vi "Coloring B-Scan Demo.vi"() -> ()   [LabVIEW 2012]
uses:
  LabVIEW/user.lib/SpectralRadar.llb/Color Enhancement Selection.ctl
  LabVIEW/user.lib/SpectralRadar.llb/Colorscheme Selection.ctl
  LabVIEW/user.lib/SpectralRadar.llb/Coloring Byteorder.ctl
  LabVIEW/user.lib/SpectralRadar.llb/Device Camera Preset Selection.ctl
  LabVIEW/user.lib/SpectralRadar.llb/Processing Parameter Int Selection.ctl
  LabVIEW/user.lib/SpectralRadar.llb/Probe Parameter Int Selection.ctl
  LabVIEW/user.lib/SpectralRadar.llb/Colored Data Export Format Selection.ctl
  LabVIEW/user.lib/SpectralRadar.llb/set Transposed Colored Scan Output.vi
  LabVIEW/user.lib/SpectralRadar.llb/set Scan Output.vi
  LabVIEW/user.lib/SpectralRadar.llb/Data.lvclass
  LabVIEW/user.lib/SpectralRadar.llb/OCT Device.lvclass
  LabVIEW/user.lib/SpectralRadar.llb/Probe.lvclass
  LabVIEW/user.lib/SpectralRadar.llb/Processing.lvclass
  LabVIEW/user.lib/SpectralRadar.llb/Raw Data.lvclass
  LabVIEW/user.lib/SpectralRadar.llb/Scan Pattern.lvclass
  LabVIEW/user.lib/SpectralRadar.llb/Coloring.lvclass
  LabVIEW/user.lib/SpectralRadar.llb/Colored Data.lvclass
  <vilib>/Analysis/NI_AALBase.lvlib
  <vilib>/Analysis/NI_AALPro.lvlib
  LabVIEW/user.lib/SpectralRadar.llb/LabVIEW Helper.lvlib
panel:
  in  "Save Button":bool
  in  "File Name":path
  in  "Display On/Off":bool
  in  "Range":dbl=1.0
  in  "Show Histogram":bool
  in  "Equalize":bool
  out "XY Graph 2":cluster{"X Values":dbl[], "Integral X":dbl[]}(graph)
  in  "Autoscale":bool
  out "XY Graph":T1(graph)
  in  "Color Table Selection":T2
  out "Averaged Frame Rate":dbl=6.134969234466553 format="%#_3g"
  out "Current Frame Rate":dbl=6.134969234466553 format="%#_3g"
  in  "Color Enhancement":T3
  in  "Boundries":cluster{sgl, sgl}(slide)={76.65738, 42.00557} scale=-20.0..120.0
  out "Image":T4(plugin-control)
  in  "stop":bool
  in  "AScans":i32=1024
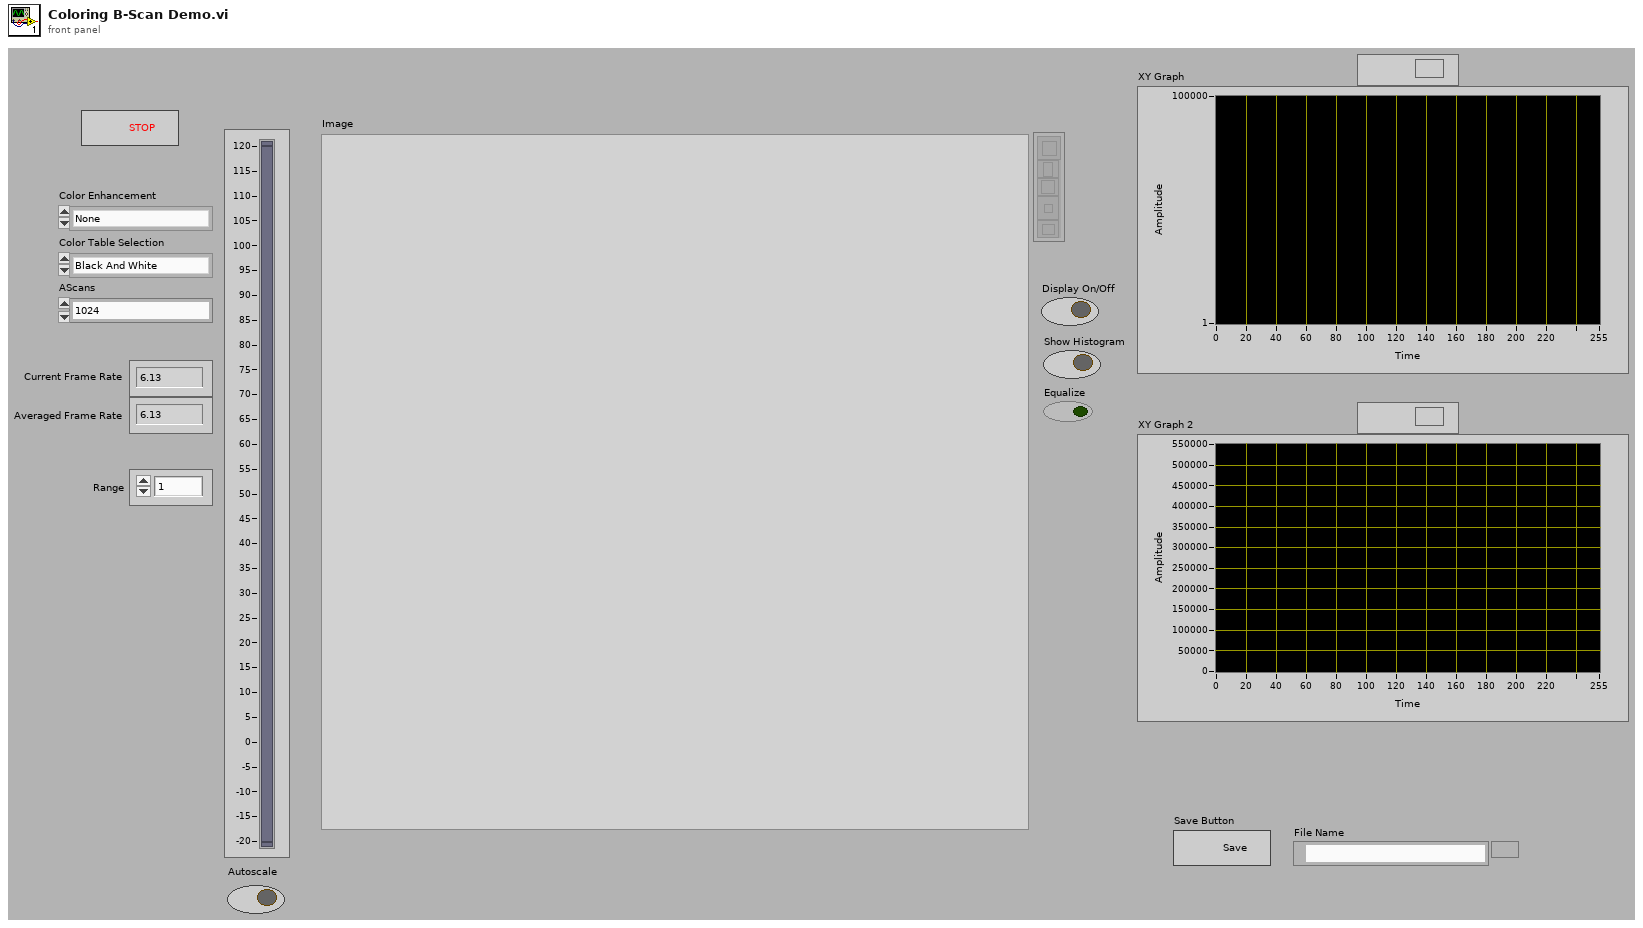
[diagram p1: front panel]
types:
  T1 = cluster{"X Values":dbl[], "Histogram: h(x)":i32[]}
  T2 = typedef "Coloring.lvclass/Colorscheme Selection.ctl" = enum16{"Black And White", "Inverted Black And White", "Color", "Black and Orange", "Black and Red", "Doppler Phase Coloring"}
  T3 = typedef "Coloring.lvclass/Color Enhancement Selection.ctl" = enum16{"None", "Sine", "Parable", "Cubic", "Square Root"}
  T4 = typedef "IMAQ Image.ctl" = refnum<image>
  T5 = typedef "Probe.lvclass/Probe Parameter Int Selection.ctl" = enum16{"Apodization Cycles", "Oversampling", "White Balance Auto", "Oversampling Slow Axis"}
  T6 = typedef "Processing.lvclass/Processing Parameter Int Selection.ctl" = enum32{"Spectrum Averaging", "A-Scan Averaging", "B-Scan Averaging", "Zero Padding", "Number of Threads", "Fourier Averaging"}
  T7 = typedef "OCT Device.lvclass/Device Camera Preset Selection.ctl" = enum16{"Default", "Preset 1", "Preset 2", "Preset 3"}
  T8 = typedef "Coloring.lvclass/Coloring Byteorder.ctl" = enum16{"RGBA32", "BGRA32", "ARGB32", ""}
  T9 = typedef "Image Type" = u32
  T10 = enum16{"Asynchronous Continuous", "Asynchronous Finite", "Synchronous"}
  T11 = typedef "Colored Data.lvclass/Colored Data Export Format Selection.ctl" = enum16{"SRM (Spectral Radar Metafile)", "RAW", "BMP", "PNG", "JPG", "PDF", "TIFF"}
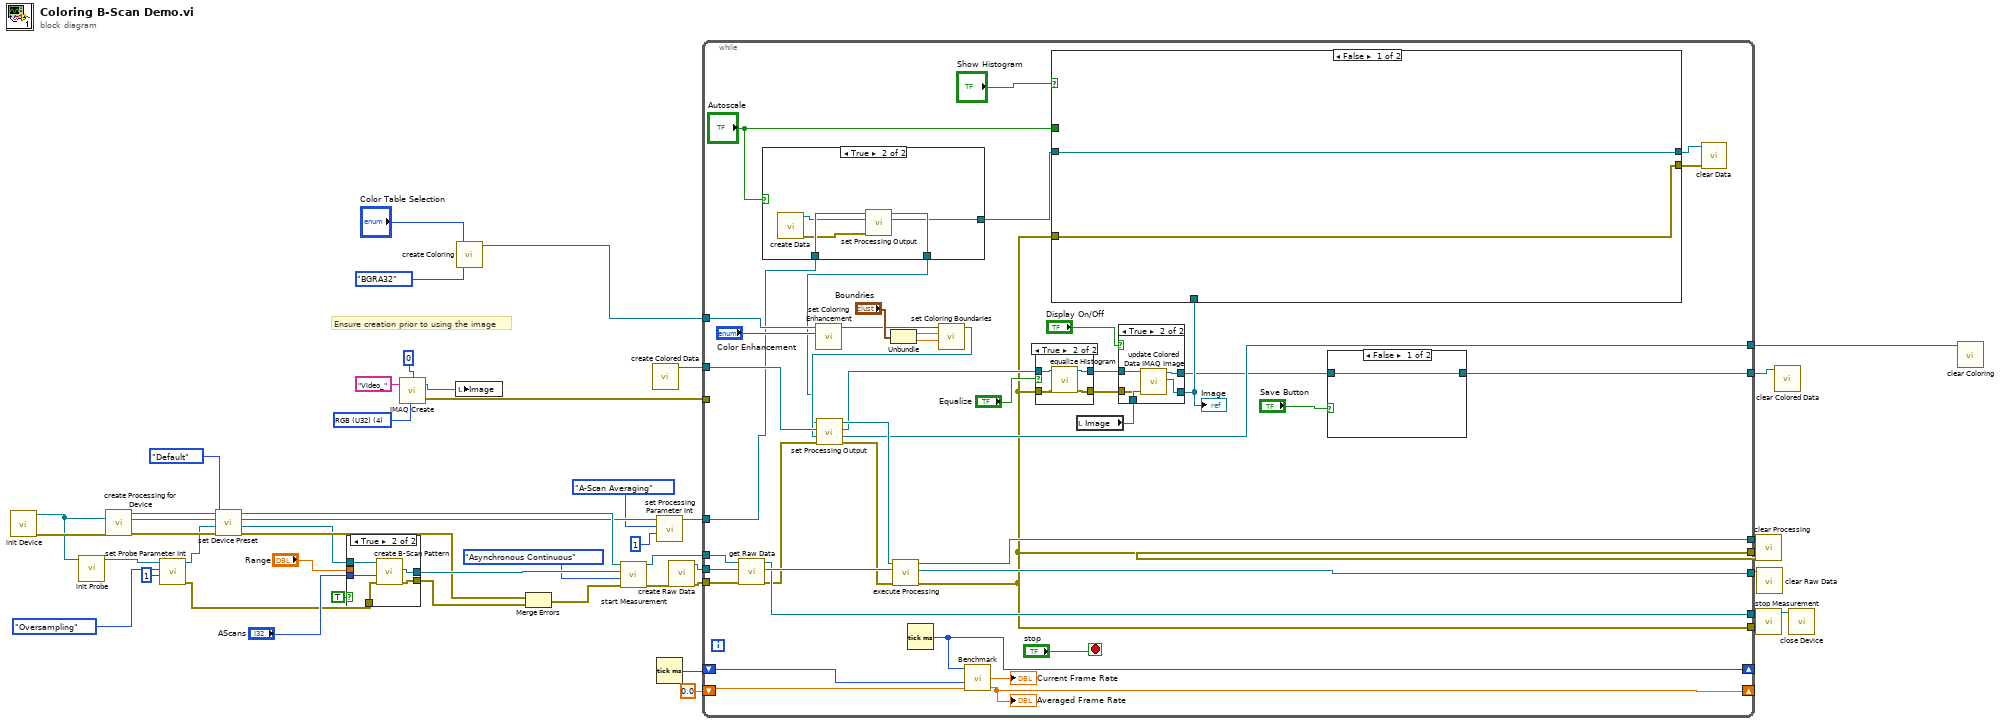
[diagram p0: block diagram]
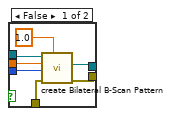
[diagram p2: hidden frame]
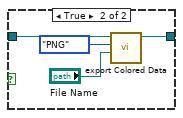
[diagram p3: hidden frame]
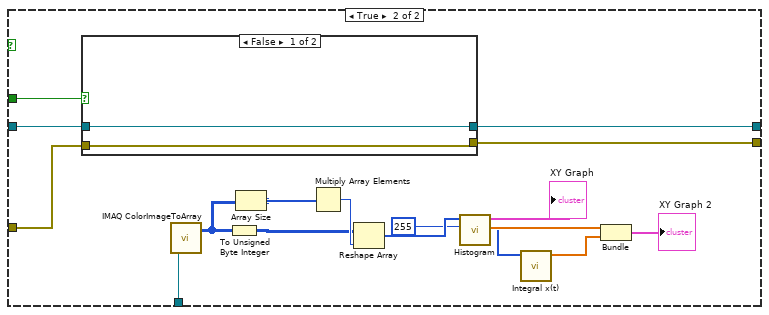
[diagram p5: hidden frame]
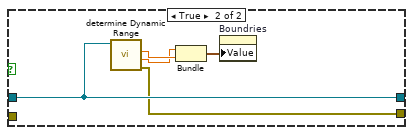
[diagram p6: hidden frame]
diagram:
  w27 = T9 4 items=["Grayscale (U8)", "Grayscale (I16)", "Grayscale (SGL)", "Complex (CSG)", "RGB (U32)", "HSL (U32)", "RGB (U64)", "Grayscale (U16)"] ("Image Type")
  # "Ensure creation prior to using the image"
  n1 = call "init Device.vi"() -> ("error out"=w46:errorcluster, "OCTDevice"=w15:refnum<class "OCT Device.lvclass">)  [unwired: 6 in]
  n2 = call "init Probe.vi"("OCT Device"=w15) -> ("GalvoControl"=w5:refnum<class "Probe.lvclass">)  [unwired: 5 in, 1 out]
  n3 = call "create Processing for Device.vi"("error in (no error)"=w46, "OCTDevice"=w15) -> ("error out"=w40:errorcluster, "Processing"=w18:refnum<class "Processing.lvclass">, "OCTDevice"=w19:refnum<class "OCT Device.lvclass">)  [unwired: 3 in]
  n4 = call "set Probe Parameter Int.vi"("Value"=1, "Probe Parameter Int"=Probe_Parameter_Int_Selection."Oversampling", "GalvoControl"=w5) -> ("error out"=w3:errorcluster, "GalvoControl"=w4:refnum<class "Probe.lvclass">)  [unwired: 3 in]
  n5 = call "set Device Preset.vi"("Numeric"=Device_Camera_Preset_Selection."Default" ("Device Camera Preset Selection"), "Probe"=w4, "Processing"=w18, "OCTDevice"=w19) -> ("Probe 2"=w14:refnum<class "Probe.lvclass">, "Processing"=w10:refnum<class "Processing.lvclass">, "OCTDevice out"=w17:refnum<class "OCT Device.lvclass">)  [unwired: 2 in, 1 out]
  n6 = case shown="True" TRUE {
    tunnel: "AScans" -> [w52 w58]
    tunnel: [w51 w57] -> w44
    tunnel: [w50 w56] -> w42
    tunnel: w3 -> [w49 w55]
    tunnel: w14 -> [w53 w54]
    tunnel: "Range" -> [w48 _]
    frame False {
      n7 = call "create Bilateral B-Scan Pattern.vi"("Rel. Shift Correction"=1.0 ("shift"), "error in (no error)"=w49, "AScans"=w52, "Range"=w48, "Probe"=w53) -> ("error out"=w50:errorcluster, "Scan Pattern"=w51:refnum<class "Scan Pattern.lvclass">)  [unwired: 2 in, 1 out]
    }
    frame True {
      n8 = call "create B-Scan Pattern.vi"("error in (no error)"=w55, "AScans"=w58, "Probe"=w54) -> ("error out"=w56:errorcluster, "Scan Pattern"=w57:refnum<class "Scan Pattern.lvclass">)  [unwired: 3 in, 1 out]
    }
  }
  n9 = call "IMAQ Create"("Border Size"=0, "Image Name"="Video_", "Image Type"=w27) -> ("New Image"=w25:T4, "error out"=w21:errorcluster)  [unwired: 2 in]
  n10 = local write "Image"(w25) -> ()
  n11 = call "create Coloring.vi"("Color Byte Order"=Coloring_Byteorder."BGRA32", "Color Table Selection"="Color Table Selection") -> ("Coloring"=w24:refnum<class "Coloring.lvclass">)  [unwired: 4 in, 1 out]
  n12 = Merge Errors(w40, w42) -> (w41:errorcluster)
  n13 = call "start Measurement.vi"("error in (no error)"=w41, "Acquisition Type"=T10."Asynchronous Continuous", "Scan Pattern"=w44, "OCTDevice"=w17) -> ("error out"=w38:errorcluster, "OCTDevice"=w31:refnum<class "OCT Device.lvclass">)  [unwired: 1 in, 1 out]
  n14 = call "create Colored Data.vi"() -> ("Colored Data"=w29:refnum<class "Colored Data.lvclass">)  [unwired: 6 in, 1 out]
  n15 = call "set Processing Parameter Int.vi"("Value"=1, "Processing Paramter Int Selection"=Processing_Parameter_Int_Selection."A-Scan Averaging", "Processing in"=w10) -> ("Processing out"=w9:refnum<class "Processing.lvclass">)  [unwired: 3 in, 1 out]
  n16 = Tick Count (ms)() -> (millisecond timer value=w23:u32)
  n17 = call "create Raw Data.vi"("error in (no error)"=w38) -> ("error out"=w37:errorcluster, "Raw Data"=w39:refnum<class "Raw Data.lvclass">)  [unwired: 5 in]
  n18 = while {
    tunnel: w39 -> [w100]
    tunnel: w31 -> [w101]
    tunnel: w37 -> [w99]
    tunnel: w9 -> [w77]
    tunnel: [w96] -> w36
    tunnel: [w95] -> w35
    tunnel: [w94] -> w33
    tunnel: [w70] -> w34
    tunnel: [w70] -> _
    tunnel: w29 -> [w80]
    tunnel: w24 -> [w84]
    shift-right: [w81] -> _
    shift-left: w23 -> [w83]
    tunnel: [w78] -> w22
    tunnel: w21 -> [_]
    shift-right: [w67] -> _
    shift-left: sgl 0.0 ("AverageFrameRate") -> [w66]
    tunnel: [w62] -> w6
    stop <- "stop" stop-if-true
    n19 = call "get Raw Data.vi"("error in (no error)"=w99, "RawData in"=w100, "OCTDevice in"=w101) -> ("error out"=w93:errorcluster, "RawData out"=w97:refnum<class "Raw Data.lvclass">, "OCTDevice out"=w94:refnum<class "OCT Device.lvclass">)  [unwired: 2 in]
    n20 = case shown="True" "Autoscale" {
      tunnel: w77 -> [w146 w151]
      tunnel: [w146 w150] -> w76
      tunnel: [_ w149] -> w75
      frame False {
      }
      frame True {
        n21 = call "create Data.vi"() -> ("error out"=w147:errorcluster, "Data"=w148:refnum<class "Data.lvclass">)  [unwired: 6 in]
        n22 = call-poly "set Processing Output.vi"("error in (no error)"=w147, "Data"=w148, "Processing"=w151) -> ("Data"=w149:refnum<class "Data.lvclass">, "Processing"=w150:refnum<class "Processing.lvclass">)  [unwired: 2 in, 1 out]
      }
    }
    n23 = call "set Coloring Enhancement.vi"("Color Enhancement"="Color Enhancement", "Coloring in"=w84) -> ("Coloring out"=w85:refnum<class "Coloring.lvclass">)  [unwired: 4 in, 1 out]
    n24 = Unbundle("Boundries") -> (w88:sgl, w87:sgl)
    n25 = Tick Count (ms)() -> (millisecond timer value=w81:u32)
    n26 = call "set Coloring Boundaries.vi"("Danymic Range High [dB]"=w87, "Dynamic Range Low [dB]"=w88, "Coloring in"=w85) -> ("Coloring out"=w79:refnum<class "Coloring.lvclass">)  [unwired: 3 in, 1 out]
    n27 = call-poly "set Processing Output.vi"("error in (no error)"=w93, "Coloring"=w79, "Colored Data"=w80, "Processing"=w76) -> ("error out"=w91:errorcluster, "Coloring"=w78:refnum<class "Coloring.lvclass">, "Colored Data"=w73:refnum<class "Colored Data.lvclass">, "Processing"=w98:refnum<class "Processing.lvclass">)
    n28 = call "execute Processing.vi"("error in (no error)"=w91, "Raw Data"=w97, "Processing"=w98) -> ("error out"=w70:errorcluster, "Raw Data"=w96:refnum<class "Raw Data.lvclass">, "Processing"=w95:refnum<class "Processing.lvclass">)  [unwired: 2 in]
    n29 = call "Benchmark.vi"("Last Frame Rate"=w66, "TimeStart"=w83, "TimeFinish"=w81) -> ("AverageFrameRate"=w67:sgl, "FrameRate"=→"Current Frame Rate":sgl)  [unwired: 1 in, 1 out]
    "Averaged Frame Rate" <- w67
    n30 = case shown="True" "Equalize" {
      tunnel: w73 -> [w140 w145]
      tunnel: [w140 w144] -> w72
      tunnel: w70 -> [w141 w143]
      tunnel: [w141 w142] -> w69
      frame False {
      }
      frame True {
        n31 = call "equalize Histogram.vi"("error in (no error)"=w143, "Colored Data in"=w145) -> ("error out"=w142:errorcluster, "Colored Data out"=w144:refnum<class "Colored Data.lvclass">)  [unwired: 4 in]
      }
    }
    n32 = local read "Image"() -> (w90:T4)
    n33 = case shown="True" "Display On/Off" {
      tunnel: w90 -> [w108 w113]
      tunnel: w72 -> [w107 w112]
      tunnel: w69 -> [_ w111]
      tunnel: [w107 w110] -> w63
      tunnel: [w108 w109] -> w64
      frame False {
      }
      frame True {
        n34 = call "update Colored Data IMAQ Image.vi"("error in (no error)"=w111, "Image in"=w113, "Colored Data"=w112) -> ("Image out"=w109:T4, "Colored Data"=w110:refnum<class "Colored Data.lvclass">)  [unwired: 2 in, 1 out]
      }
    }
    "Image" <- w64
    n35 = case shown="False" "Show Histogram" {
      tunnel: w64 -> [_ w132]
      tunnel: w75 -> [w115 w125]
      tunnel: "Autoscale" -> [_ w124]
      tunnel: w70 -> [w114 w118]
      tunnel: [w115 w117] -> w60
      tunnel: [w114 w116] -> w59
      frame False {
      }
      frame True {
        n36 = case shown="False" w124 {
          tunnel: w118 -> [w134 _]
          tunnel: w125 -> [w133 w136]
          tunnel: [w133 w136] -> w117
          tunnel: [w134 w135] -> w116
          frame False {
          }
          frame True {
            n37 = call "determine Dynamic Range.vi"("Data in"=w136) -> ("error out"=w135:errorcluster, "High"=w137:sgl, "Low"=w138:sgl)  [unwired: 3 in, 1 out]
            n38 = Bundle("High"=w137, "Low"=w138) -> (w139:cluster{"High":sgl, "Low":sgl})  [unwired: 1 in]
            n39 = property on="Boundries" class="Slide (strict)"("Value"=w139) -> ()  [unwired: 2 in, 2 out]
          }
        }
        n40 = call "IMAQ ColorImageToArray"("Image"=w132) -> ("Image Pixels (U32)"=w127:u32[][])  [unwired: 3 in, 2 out]
        n41 = To Unsigned Byte Integer(number=w127) -> (unsigned 8bit integer=w126:u8[][])
        n42 = Array Size(array=w127) -> (size(s)=w129:i32[])
        n43 = Multiply Array Elements(1:w129) -> (0:w128:i32)
        n44 = Reshape Array(w126, w128) -> (w131:u8[])
        n45 = call <vilib>:"Histogram.vi"("intervals"=255, "X"=w131) -> ("X Values"=w122:dbl[], "Histogram: h(x)"=w121:i32[], "Histogram Graph"=→"XY Graph":T1)  [unwired: 6 in, 1 out]
        n46 = call <vilib>:"Integral x(t).vi"("X"=w121) -> ("Integral X"=w120:dbl[])  [unwired: 9 in, 1 out]
        n47 = Bundle("X Values"=w122, "Integral X"=w120) -> (→"XY Graph 2":cluster{"X Values":dbl[], "Integral X":dbl[]})  [unwired: 1 in]
      }
    }
    n48 = case shown="False" "Save Button" {
      tunnel: w63 -> [w102 w106]
      tunnel: [w102 w105] -> w62
      frame False {
      }
      frame True {
        n49 = call "export Colored Data.vi"("File Name"="File Name", "Colored Data Export Format Selection"=Colored_Data_Export_Format_Selection."PNG", "Colored Data in"=w106) -> ("Colored Data out"=w105:refnum<class "Colored Data.lvclass">)  [unwired: 3 in, 1 out]
      }
    }
    n50 = call "clear Data.vi"("error in (no error)"=w59, "Data"=w60) -> ()  [unwired: 5 in, 1 out]
  }
  n51 = call "clear Processing.vi"("error in (no error)"=w34, "Processing"=w35) -> ()  [unwired: 5 in, 1 out]
  n52 = call "stop Measurement.vi"("OCTDevice"=w33) -> ("OCTDevice"=w32:refnum<class "OCT Device.lvclass">)  [unwired: 5 in, 1 out]
  n53 = call "clear Raw Data.vi"("Raw Data"=w36) -> ()  [unwired: 6 in, 1 out]
  n54 = call "clear Colored Data.vi"("Colored Data"=w6) -> ()  [unwired: 6 in, 1 out]
  n55 = call "close Device.vi"("OCTDevice"=w32) -> ()  [unwired: 6 in, 1 out]
  n56 = call "clear Coloring.vi"("Coloring"=w22) -> ()  [unwired: 6 in, 1 out]
